vi "pmu_Analog Digit Scale.vi"(6 "nominal frequency":enum16{"50 Hz", "60 Hz"}(ring), 8 "dfreq in":sgl, 9 "freq in":sgl, 10 "analogs in":sgl[](array[numeric]), 11 "format":u16) -> (0 "freq out of range":bool, 1 "analog out of range":bool, 2 "analogs byte array":u8[](array[numeric]), 3 "dfreq byte array":u8[](array[numeric]), 4 "df/dt out of range":bool, 5 "freq byte array":u8[](array[numeric]))   [LabVIEW 2013, in "NI_EP_PMU.lvlib"]
uses:
  <vilib>/addons/Electrical Power/PMU/NI_EP_PMU.lvlib
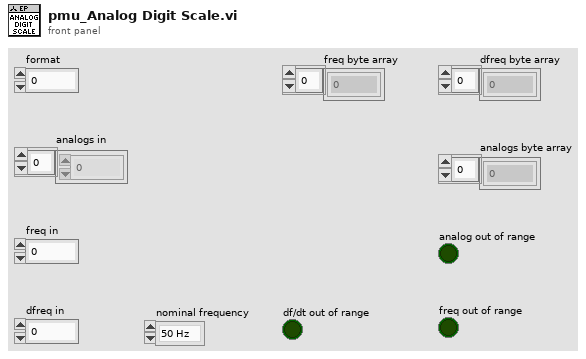
[diagram p1: front panel]
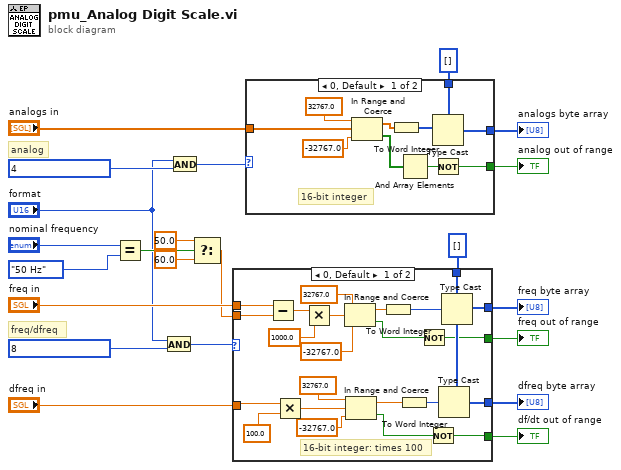
[diagram p0: block diagram]
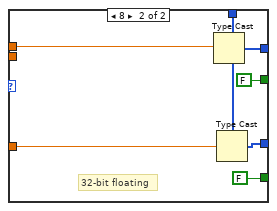
[diagram p2: hidden frame]
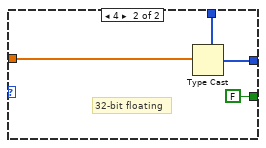
[diagram p3: hidden frame]
diagram:
  # "freq/dfreq"
  # "analog"
  n1 = Equal?(x="nominal frequency", y=enum16{"50 Hz", "60 Hz"}."50 Hz" ("nominal frequency 2")) -> (x = y?=w8:bool)
  n2 = And(x="format", y=u16 8 ("x")) -> (x .and. y?=w19:u16)
  n3 = And(x="format", y=u16 4 ("x")) -> (x .and. y?=w20:u16)
  n4 = Select(t=50.0, s=w8, f=60.0) -> (s? t:f=w5:dbl)
  n5 = case shown="0, Default" w19 {
    tunnel: "freq in" -> [w41 w49]
    tunnel: "dfreq in" -> [w29 w46]
    tunnel: u8[] [] ("appended array") -> [w44 w51]
    tunnel: [w45 w52] -> w12
    tunnel: [w42 w50] -> w11
    tunnel: w5 -> [w40 _]
    tunnel: [w25 FALSE] -> w4
    tunnel: [w24 FALSE] -> w3
    frame 0, Default {
      # "16-bit integer: times 100"
      n6 = Subtract(x=w41, y=w40) -> (x-y=w39:dbl)
      n7 = Multiply(x=w29, y=sgl 100.0) -> (x*y=w27:sgl)
      n8 = Multiply(x=w39, y=1000.0) -> (x*y=w37:dbl)
      n9 = In Range and Coerce(upper limit=32767.0 ("y"), x=w37, lower limit=-32767.0 ("y")) -> (coerced(x)=w34:dbl, In Range?=w26:bool)
      n10 = In Range and Coerce(upper limit=sgl 32767.0 ("y"), x=w27, lower limit=sgl -32767.0 ("y")) -> (coerced(x)=w30:sgl, In Range?=w23:bool)
      n11 = To Word Integer(number=w34) -> (16bit integer=w33:i16)
      n12 = To Word Integer(number=w30) -> (16bit integer=w43:i16)
      n13 = Not(x=w26) -> (.not. x?=w25:bool)
      n14 = Not(x=w23) -> (.not. x?=w24:bool)
      n15 = Type Cast(type=w44, x=w43) -> (*(type *) &x=w42:u8[])
      n16 = Type Cast(type=w44, x=w33) -> (*(type *) &x=w45:u8[])
    }
    frame 8 {
      # "32-bit floating"
      n17 = Type Cast(type=w51, x=w49) -> (*(type *) &x=w52:u8[])
      n18 = Type Cast(type=w51, x=w46) -> (*(type *) &x=w50:u8[])
    }
  }
  "freq byte array" <- w12
  "dfreq byte array" <- w11
  "freq out of range" <- w4
  "df/dt out of range" <- w3
  n19 = case shown="0, Default" w20 {
    tunnel: "analogs in" -> [w57 w65]
    tunnel: u8[] [] ("appended array") -> [w61 w66]
    tunnel: [w60 w64] -> w16
    tunnel: [w53 FALSE] -> w2
    frame 0, Default {
      # "16-bit integer"
      n20 = In Range and Coerce(upper limit=sgl 32767.0 ("y"), x=w57, lower limit=sgl -32767.0 ("y")) -> (coerced(x)=w56:sgl[], In Range?=w54:bool[])
      n21 = To Word Integer(number=w56) -> (16bit integer=w62:i16[])
      n22 = And Array Elements(Boolean array=w54) -> (logical AND=w55:bool)
      n23 = Type Cast(type=w61, x=w62) -> (*(type *) &x=w60:u8[])
      n24 = Not(x=w55) -> (.not. x?=w53:bool)
    }
    frame 4 {
      # "32-bit floating"
      n25 = Type Cast(type=w66, x=w65) -> (*(type *) &x=w64:u8[])
    }
  }
  "analogs byte array" <- w16
  "analog out of range" <- w2
